vi "New Message Buffer.vi"(8 "error in":errorcluster, 9 "MessageData (0x0000)":u16[](array[numeric]) format="%04x", 10 "MessageBuffer configuration":T1={"bufferMaxEntries"=1, "bufferType"=0, "eventLogOnEmptyOrFull"=FALSE, "eventLogOnHalf"=FALSE} {"bufferType" items=["FIFO", "Circular"]}, 11 "name":string="CoreName") -> (0 "error out":errorcluster, 1 "ID out":i32, 3 "new messageBuffer":refnum<k24>)   [LabVIEW 2020, in "Ballard_1553_Hardware_ni.lvlib"]
uses:
  Ballard_1553_Hardware_ni.lvlib
  C:/Users/Administrator/Desktop/GIT/Ballard-MIL-STD-1553-Custom-Device/Source/System Explorer/SubVIs/Parse XML Ballard/1.2/BTIXML_SerDes.dll
  Ballard-MIL-STD-1553-Custom-Device/Source/System Explorer/SubVIs/Parse XML Ballard/1.2/BTIXML_SerDes.dll
  _typedefs/MessageBuffer_type.ctl
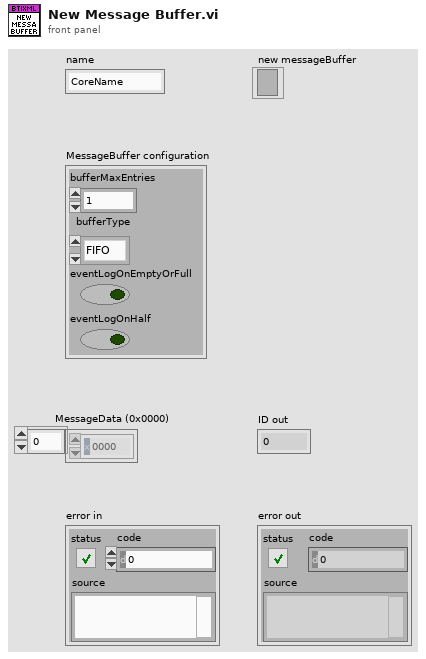
[diagram p1: front panel]
types:
  T1 = typedef "Ballard_1553_Hardware_ni.lvlib/MessageBuffer_type.ctl" = cluster{"bufferMaxEntries":i32, "bufferType":i32, "eventLogOnEmptyOrFull":bool, "eventLogOnHalf":bool}
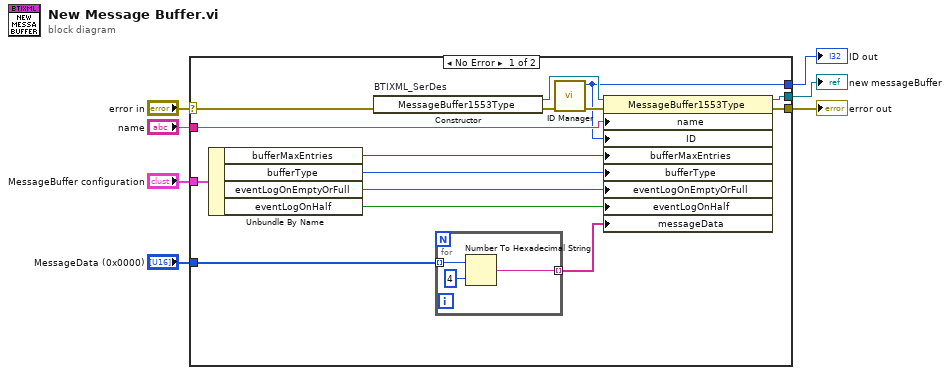
[diagram p0: block diagram]
diagram:
  n1 = case shown="No Error" "error in" {
    selector: "error in" -> [w21 w26]
    tunnel: [w20 w26] -> w6
    tunnel: [w19 _] -> w4
    tunnel: "name" -> [w18 _]
    tunnel: "MessageBuffer configuration" -> [w15 _]
    tunnel: "MessageData (0x0000)" -> [w10 _]
    tunnel: [w8 _] -> w1
    frame No Error {
      n2 = Unbundle By Name(w15) -> ("bufferMaxEntries"=w14:i32, "bufferType"=w13:i32, "eventLogOnEmptyOrFull"=w12:bool, "eventLogOnHalf"=w11:bool)
      n3 = constructor on="BTIXML_SerDes" class="MessageBuffer1553Type"(error in=w21) -> (reference out=w22:refnum<k24>, error out=w17:errorcluster)  [unwired: 2 in, 1 out]
      n4 = for {
        tunnel: w10 -> [w25] mode=indexing
        tunnel: [w24] -> w9 mode=indexing
        n5 = Number To Hexadecimal String(1:i16 4 ("width (-)"), 2:w25) -> (0:w24:string)
      }
      n6 = call "ID Manager.vi"("error in"=w17) -> ("error out"=w16:errorcluster, "ID out"=w8:i32)  [unwired: 9 in]
      n7 = property class="MessageBuffer1553Type"(reference=w22, error in=w16, "name"=w18, "ID"=w8, "bufferMaxEntries"=w14, "bufferType"=w13, "eventLogOnEmptyOrFull"=w12, "eventLogOnHalf"=w11, "messageData"=w9) -> (reference out=w19:refnum<k24>, error out=w20:errorcluster)
    }
    frame Error {
    }
  }
  "error out" <- w6
  "new messageBuffer" <- w4
  "ID out" <- w1
